vi "Get_folder_and_filenames.vi"(0 "file path (dialog if empty)":path) -> (1 "Folders":path[](array[path]), 2 "Files":path[](array[path]))   [LabVIEW 2020]
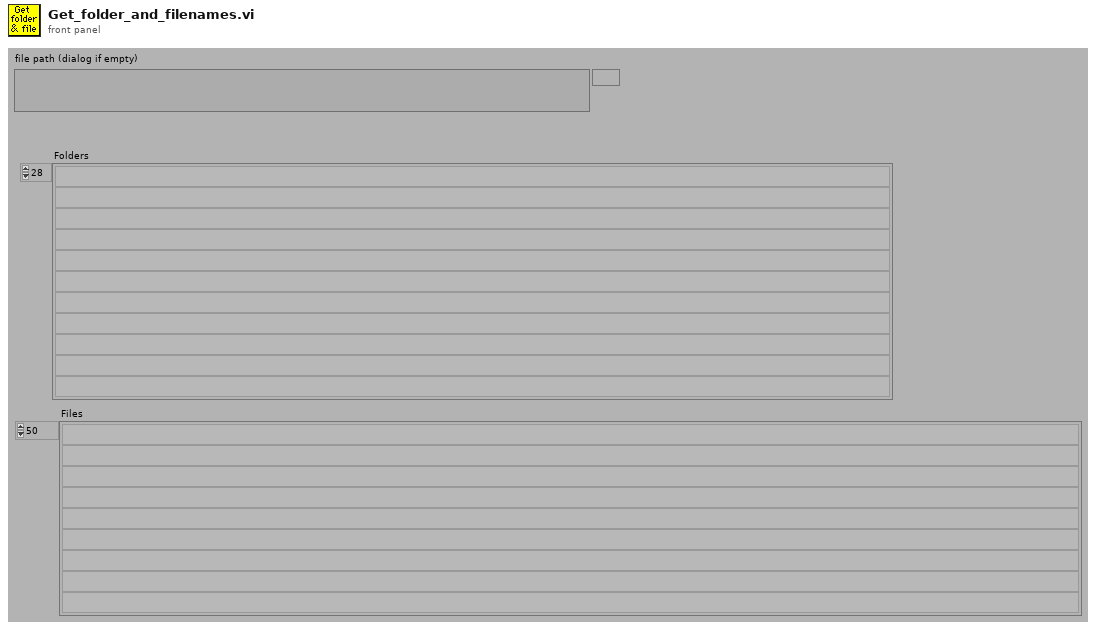
[diagram p1: front panel]
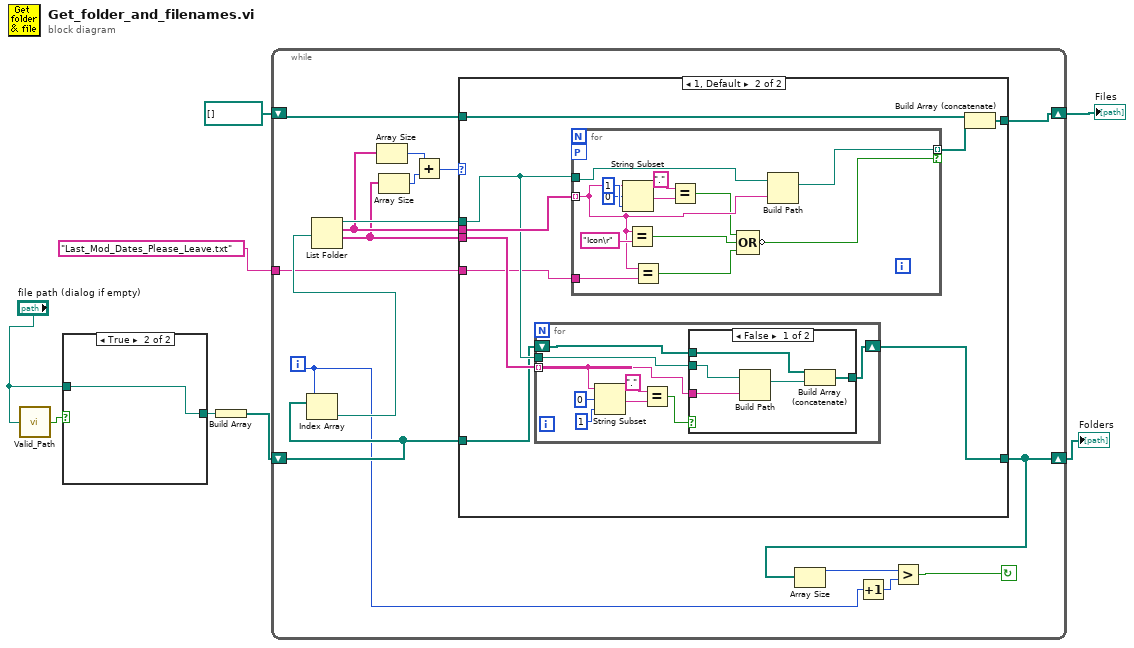
[diagram p0: block diagram]
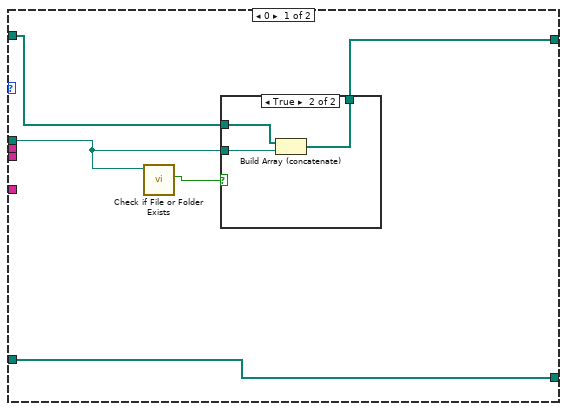
[diagram p2: hidden frame]
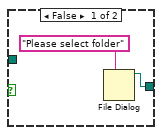
[diagram p5: hidden frame]
diagram:
  n1 = call "Valid_Path.vi"("Filename"="file path (dialog if empty)") -> ("Valid Path?"=w1:bool)
  n2 = case shown="True" w1 {
    tunnel: [w10 w11] -> w7
    tunnel: "file path (dialog if empty)" -> [_ w11]
    frame False {
      n3 = File Dialog(7:"Please select folder" ("prompt")) -> (3:w10:path)  [unwired: 1 in, 8 out]
    }
    frame True {
    }
  }
  n4 = Build Array(w7) -> (w6:path[])
  n5 = while {
    shift-left: w6 -> [w25]
    shift-right: [w14] -> w8
    tunnel: "Last_Mod_Dates_Please_Leave.txt" -> [w24]
    shift-right: [w22] -> w3
    shift-left: path[] [] -> [w23]
    i -> [w12]
    stop <- w13 continue-if-true
    n6 = Index Array(array=w25, index=w12) -> (element=w27:path)
    n7 = List Folder(path=w27) -> (path out=w26:path, filenames=w21:string[], folder names=w20:string[])  [unwired: 1 in, 3 out]
    n8 = Array Size(array=w21) -> (size(s)=w18:i32)
    n9 = Array Size(array=w20) -> (size(s)=w19:i32)
    n10 = Add(x=w18, y=w19) -> (x+y=w17:i32)
    n11 = case shown="1, Default" w17 {
      tunnel: w21 -> [_ w45]
      tunnel: w26 -> [w31 w44]
      tunnel: w20 -> [_ w43]
      tunnel: w25 -> [w28 w42]
      tunnel: [w28 w41] -> w14
      tunnel: w24 -> [_ w40]
      tunnel: w23 -> [w29 w39]
      tunnel: [w32 w37] -> w22
      frame 0 {
        n12 = call <vilib>:"Check if File or Folder Exists.vi"("path"=w31) -> ("file or folder exists?"=w30:bool)  [unwired: 8 in, 2 out]
        n13 = case shown="True" w30 {
          tunnel: [w33 w36] -> w32
          tunnel: w31 -> [_ w35]
          tunnel: w29 -> [w33 w34]
          frame False {
          }
          frame True {
            n14 = Build Array (concatenate)(w34, w35) -> (w36:path[])
          }
        }
      }
      frame 1, Default {
        n15 = for {
          tunnel: w44 -> [w49]
          tunnel: w43 -> [w48] mode=indexing
          shift-right: [w46] -> w41
          shift-left: w42 -> [w47]
          n16 = String Subset(string=w48, offset (0)=0, length (rest)=1 ("length")) -> (substring=w53:string)
          n17 = Equal?(x=".", y=w53) -> (x = y?=w50:bool)
          n18 = case shown="False" w50 {
            tunnel: w48 -> [w59 _]
            tunnel: w49 -> [w58 _]
            tunnel: w47 -> [w57 w60]
            tunnel: [w55 w60] -> w46
            frame False {
              n19 = Build Path(base path=w58, name or relative path=w59) -> (appended path=w56:path)
              n20 = Build Array (concatenate)(w57, w56) -> (w55:path[])
            }
            frame True {
            }
          }
        }
        n21 = for {
          tunnel: w44 -> [w69]
          tunnel: w45 -> [w66] mode=indexing
          tunnel: [w67] -> w38 mode=indexing if=w61
          tunnel: w40 -> [w65]
          workers-P: _ -> [_]
          n22 = String Subset(string=w66, offset (0)=0, length (rest)=1 ("length")) -> (substring=w71:string)
          n23 = Equal?(x=w66, y="Icon\r") -> (x = y?=w63:bool)
          n24 = Equal?(x=w66, y=w65) -> (x = y?=w62:bool)
          n25 = Equal?(x=".", y=w71) -> (x = y?=w64:bool)
          n26 = Compound Arithmetic op=OR(w64, w63, w62) -> (invert w61:bool)
          n27 = Build Path(base path=w69, name or relative path=w66) -> (appended path=w67:path)
        }
        n28 = Build Array (concatenate)(w39, w38) -> (w37:path[])
      }
    }
    n29 = Array Size(array=w14) -> (size(s)=w16:i32)
    n30 = Increment(x=w12) -> (x+1=w15:i32)
    n31 = Greater?(x=w16, y=w15) -> (0:w13:bool)
  }
  "Folders" <- w8
  "Files" <- w3
